vi "PRIME Detector Pipeline Check Status for New Files.vi"(5 "Observation":T2={"Priority"=0, "ID"="", "Observer"="", "Obj Name"="", "Obj Type"="", "RA and DEC String"={"RA"="HH:MM:SS.nnn", "DEC"="DEG:arcmin:arcsec.nn"}, "Filter Wheel 1"="", "Filter Wheel 2"="", "Integration Time"=0.0, "Observation Status"=enum."Error", "Offsets"={"RA"=0.0, "DEC"=0.0, "ROT"=0.0}, "Images"=0, "Dither Options"={"Dither"=enum."None", "Dither Radius"=0.0, "Dither Points"=0, "Dither Phase"=0.0}, "Comment 1"="", "Comment 2"=""}, 7 "Detector Config":T7={"Detector"=0, "Offsets"=[[0, 0, 0, 0, 0, 0, 0, 0, 0, 0, 0, 0, 0, 0, 0, 0, 0, 0, 0, 0, 0, 0, 0, 0, 0, 0, 0, 0, 0, 0, 0, 0]], "Detector Computer"={"Machine"="192.168.121.11", "Password"="rSL!nux23456", "FITS File Path"="", "Port"=44444, "Header Path"="", "Name"=""}, "FITS hdr template0"=path "", "FITS hdr template1"=path "", "FITS Data File Path"=path "", "FITS Detector Settings"={"Exp Time Short"=0.0, "# of Frames"=0.0, "Exp Time Long"=0.0, "# of Groups"=0.0, "Object Name"="", "Object"="", "Obs Type"="", "Image Type"="", "Observer"="", "Observer Affiliation"=""}, "Sim Folder"=path "", "Integration Mode"=enum."SSR", "Integration Time"=0.0, "Frame Int Time"=0.0} {"Offsets" format="%04x"; "Detector" items=["0", "1", "2"]}, 8 "error in (no error)":errorcluster, 10 "Status":T1, 11 "Map in":map{string, T11}(c390)) -> (0 "error out":errorcluster, 3 "Map out":map{string, T11}(c390))   [LabVIEW 2024]
uses:
  Detector Image typedef cluster.ctl
  RIMAS Detector Config.ctl
  RIMAS Detector Server Config.ctl
  RIMAS Observation Config.ctl
  Detector enum Detector Integration Mode.ctl
  typedefs/CC cluster Observation.ctl
  Observation Queue/CC enum Observation Status.ctl
  Telescope/CC cluster Telescope Offsets.ctl
  typedefs/CC cluster Observation Dither Options.ctl
  typedefs/CC enum Dither Selection.ctl
  PRIME Detector cluster Status.ctl
  Detector Class.lvclass
panel:
  # "sec"
  # "sec"
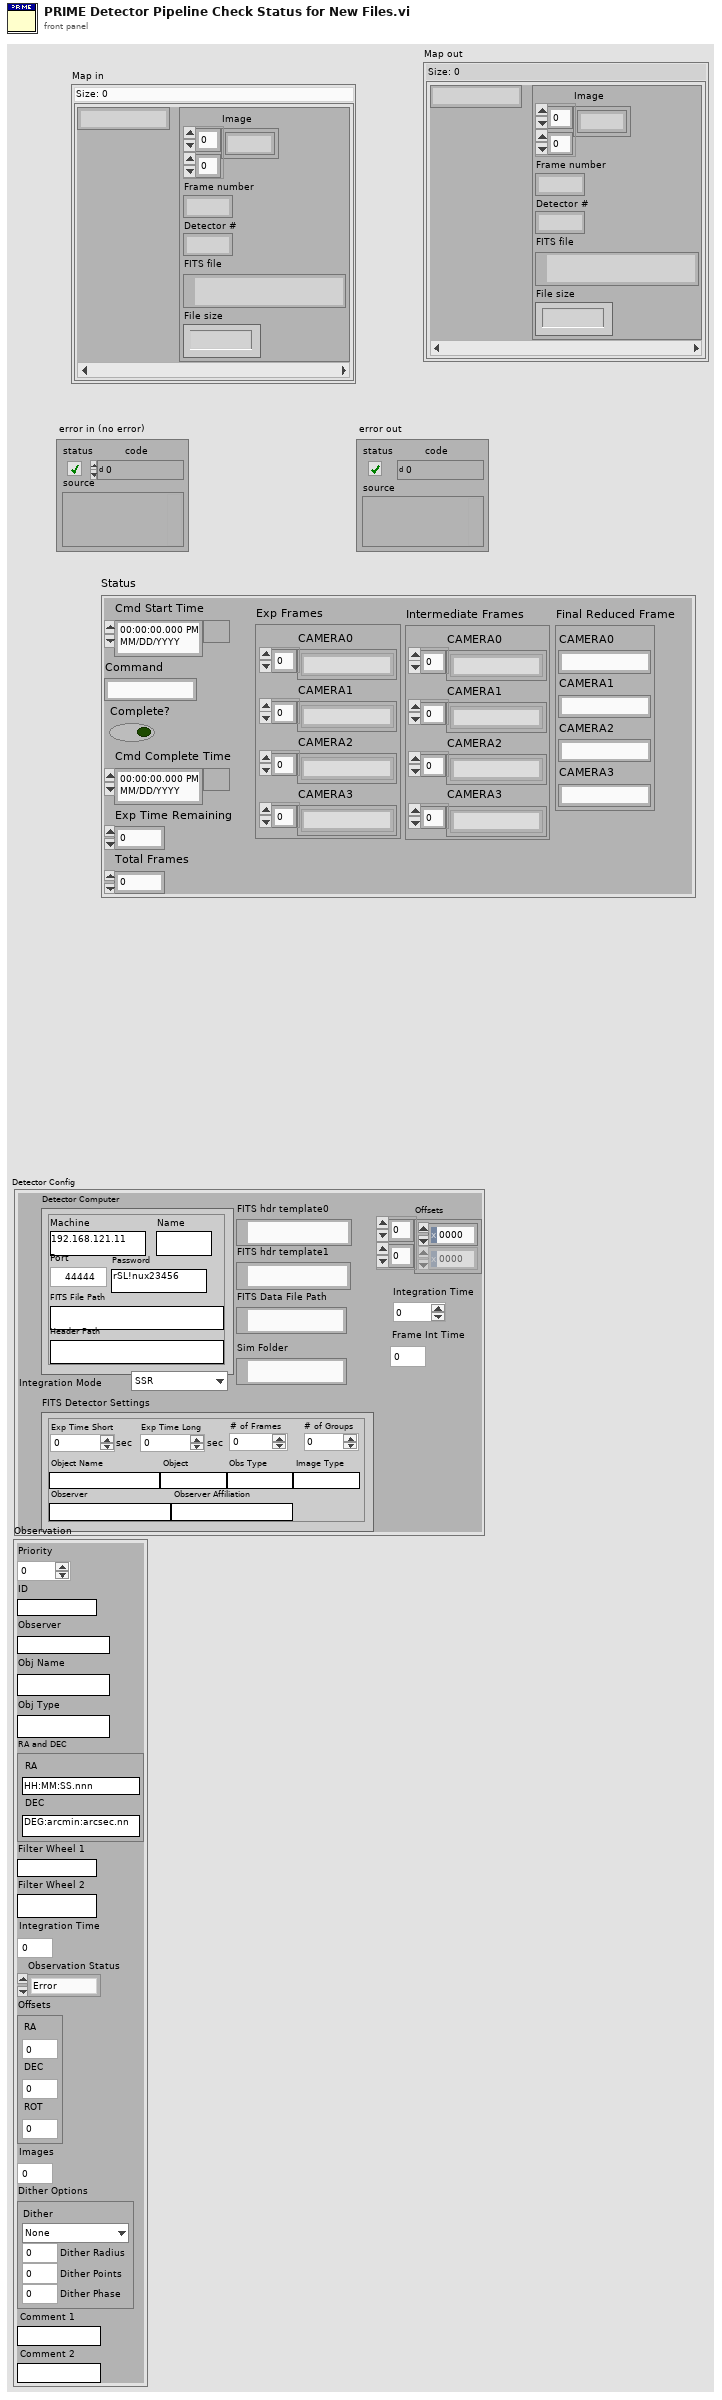
[diagram p1: front panel]
types:
  T1 = typedef "PRIME Detector cluster Status.ctl" = cluster{"Cmd Start Time":timestamp, "Command":string, "Complete?":bool, "Cmd Complete Time":timestamp, "Exp Time Remaining":dbl, "Total Frames":i32, "Exp Frames":cluster{"CAMERA0":string[], "CAMERA1":string[], "CAMERA2":string[], "CAMERA3":string[]}, "Intermediate Frames":cluster{"CAMERA0":string[], "CAMERA1":string[], "CAMERA2":string[], "CAMERA3":string[]}, "Final Reduced Frame":cluster{"CAMERA0":string, "CAMERA1":string, "CAMERA2":string, "CAMERA3":string}}
  T2 = typedef "CC cluster Observation.ctl" = cluster{"Priority":i32, "ID":string, "Observer":string, "Obj Name":string, "Obj Type":string, "RA and DEC String":cluster{"RA":string, "DEC":string}, "Filter Wheel 1":string, "Filter Wheel 2":string, "Integration Time":dbl, "Observation Status":T3, "Offsets":T4, "Images":i32, "Dither Options":T5, "Comment 1":string, "Comment 2":string}
  T3 = typedef "CC enum Observation Status.ctl" = enum16{"Ready", "Running", "Done", "Error"}
  T4 = typedef "CC cluster Telescope Offsets.ctl" = cluster{"RA":dbl, "DEC":dbl, "ROT":dbl}
  T5 = typedef "CC cluster Observation Dither Options.ctl" = cluster{"Dither":T6, "Dither Radius":dbl, "Dither Points":i32, "Dither Phase":dbl}
  T6 = typedef "CC enum Dither Selection.ctl" = enum16{"None", "Circle", "Random"}
  T7 = typedef "RIMAS Detector Config.ctl" = cluster{"Detector":u16, "Offsets":u16[][], "Detector Computer":T8, "FITS hdr template0":path, "FITS hdr template1":path, "FITS Data File Path":path, "FITS Detector Settings":T9, "Sim Folder":path, "Integration Mode":T10, "Integration Time":dbl, "Frame Int Time":dbl}
  T8 = typedef "RIMAS Detector Server Config.ctl" = cluster{"Machine":string, "Password":string, "FITS File Path":string, "Port":u16, "Header Path":string, "Name":string}
  T9 = typedef "RIMAS Observation Config.ctl" = cluster{"Exp Time Short":dbl, "# of Frames":dbl, "Exp Time Long":dbl, "# of Groups":dbl, "Object Name":string, "Object":string, "Obs Type":string, "Image Type":string, "Observer":string, "Observer Affiliation":string}
  T10 = typedef "Detector enum Detector Integration Mode.ctl" = enum16{"SSR", "CDS", "MEAN", "MEDIAN", "MODE", "MIIN", "MAX"}
  T11 = typedef "Detector Class.lvclass/Detector Image typedef cluster.ctl" = cluster{"Image":sgl[][], "Frame number":i32, "Detector #":u16, "FITS file":path, "File size":i64}
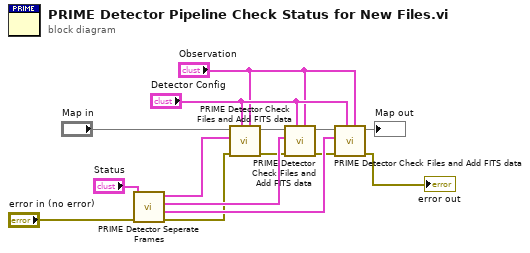
[diagram p0: block diagram]
diagram:
  n1 = call "PRIME Detector Seperate Frames.vi"("error in (no error)"="error in (no error)", "Status"="Status") -> ("error out"=w7:errorcluster, "Final Frames"=w11:cluster{string[]}[], "Inter Frames"=w12:cluster{"CAMERA3":string[]}[], "Exp Frames"=w15:cluster{"CAMERA3":string[]}[])  [unwired: 6 in]
  n2 = call "PRIME Detector Check Files and Add FITS data.vi"("Observation"="Observation", "Detector Config"="Detector Config", "error in (no error)"=w7, "Image Array"=w15, "Map in"="Map in") -> ("error out"=w6:errorcluster, "Map out"=w14:map{string, T11})  [unwired: 5 in]
  n3 = call "PRIME Detector Check Files and Add FITS data.vi"("Observation"="Observation", "Detector Config"="Detector Config", "error in (no error)"=w6, "Image Array"=w12, "Map in"=w14) -> ("error out"=w5:errorcluster, "Map out"=w13:map{string, T11})  [unwired: 5 in]
  n4 = call "PRIME Detector Check Files and Add FITS data.vi"("Observation"="Observation", "Detector Config"="Detector Config", "error in (no error)"=w5, "Image Array"=w11, "Map in"=w13) -> ("error out"=→"error out":errorcluster, "Map out"=→"Map out":map{string, T11})  [unwired: 5 in]
